vi "Create Level String.vi"(8 "Error In":errorcluster, 11 "Level":T1) -> (0 "Error Out":errorcluster, 3 "String":string)   [LabVIEW 2017, in "Toolkit.lvlib"]
uses:
  Toolkit.lvlib
  Controls/Tag.ctl
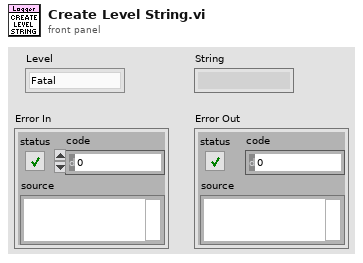
[diagram p1: front panel]
types:
  T1 = typedef "Toolkit.lvlib/Tag.ctl" = enum16{"Fatal", "Error", "Warn", "Info", "Debug", "Trace"}
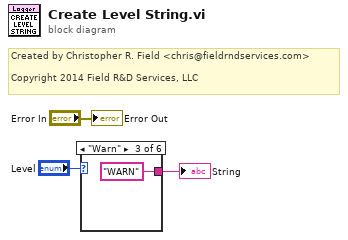
[diagram p0: block diagram]
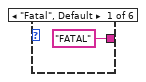
[diagram p2: hidden frame]
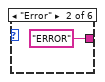
[diagram p3: hidden frame]
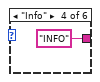
[diagram p4: hidden frame]
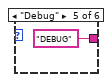
[diagram p5: hidden frame]
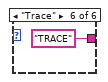
[diagram p6: hidden frame]
diagram:
  # "Created by Christopher R. Field <chris@fieldrndservices.com>\n\nCopyright 2014 Field R&D Services, LLC"
  n1 = case shown="\"Warn\"" "Level" {
    tunnel: ["FATAL" "ERROR" "WARN" "INFO" "DEBUG" "TRACE"] -> w2
    frame "Fatal", Default {
    }
    frame "Error" {
    }
    frame "Warn" {
    }
    frame "Info" {
    }
    frame "Debug" {
    }
    frame "Trace" {
    }
  }
  "String" <- w2
  "Error Out" <- "Error In"
